vi "Hex_to_Binary.vi"(6 "error in (no error)":errorcluster, 9 "Hexadecimal String":string) -> (0 "error out":errorcluster, 2 "add 0's' String":string, 3 "Binary String":string)   [LabVIEW 2018]
panel:
  out "Number in Binary display format":u64 format="%064b"
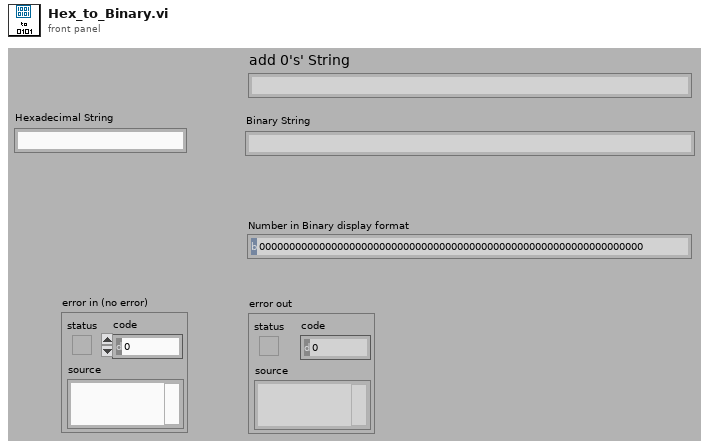
[diagram p1: front panel]
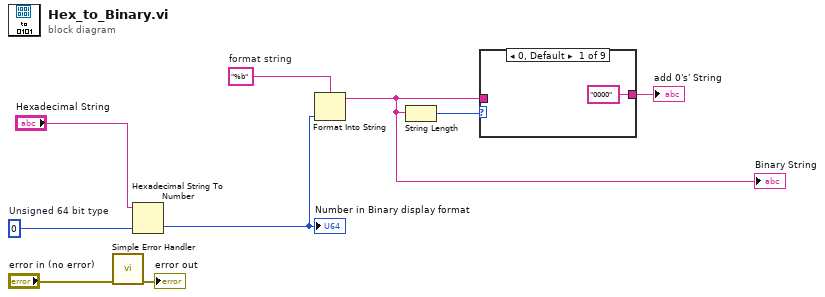
[diagram p0: block diagram]
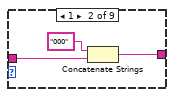
[diagram p2: hidden frame]
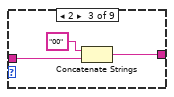
[diagram p3: hidden frame]
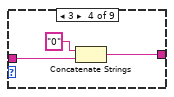
[diagram p4: hidden frame]
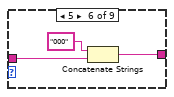
[diagram p6: hidden frame]
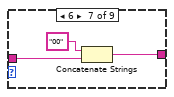
[diagram p7: hidden frame]
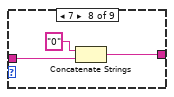
[diagram p8: hidden frame]
diagram:
  w8 = u64 0  # Unsigned 64 bit type
  w9 = "%b"  # format string
  n1 = call <vilib>:"Simple Error Handler.vi"("error in (no error)"="error in (no error)") -> ("error out"=→"error out":errorcluster)  [unwired: 4 in, 4 out]
  n2 = Hexadecimal String To Number(string="Hexadecimal String", default (0uL)=w8) -> (number=w1:u64)  [unwired: 1 in, 1 out]
  "Number in Binary display format" <- w1
  n3 = Format Into String "Format Into String"(format string=w9, w1) -> (resulting string=w3:string)  [unwired: 2 in, 1 out]
  "Binary String" <- w3
  n4 = String Length(string=w3) -> (length=w4:i32)
  n5 = case shown="0, Default" w4 {
    tunnel: w3 -> [_ w12 w15 w18 w20 w22 w25 w28 w30]
    tunnel: ["0000" w13 w14 w17 w20 w21 w24 w27 w30] -> w2
    frame 0, Default {
    }
    frame 1 {
      n6 = Concatenate Strings("000" ("string"), w12) -> (w13:string)
    }
    frame 2 {
      n7 = Concatenate Strings("00" ("string"), w15) -> (w14:string)
    }
    frame 3 {
      n8 = Concatenate Strings("0" ("string"), w18) -> (w17:string)
    }
    frame 4 {
    }
    frame 5 {
      n9 = Concatenate Strings("000" ("string"), w22) -> (w21:string)
    }
    frame 6 {
      n10 = Concatenate Strings("00" ("string"), w25) -> (w24:string)
    }
    frame 7 {
      n11 = Concatenate Strings("0" ("string"), w28) -> (w27:string)
    }
    frame 8 {
    }
  }
  "add 0's' String" <- w2
